vi "Describe Boolean Failure.vi"(1 "Expected":bool, 2 "Got":bool) -> (0 "Failure Description":string)   [LabVIEW 2013]
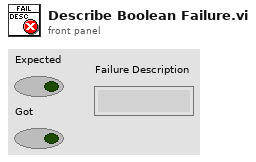
[diagram p1: front panel]
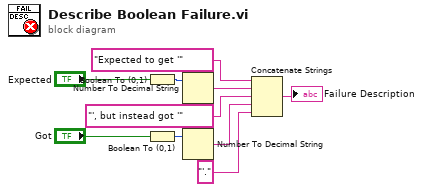
[diagram p0: block diagram]
diagram:
  n1 = Boolean To (0,1)(Boolean="Expected") -> (0, 1=w7:i16)
  n2 = Boolean To (0,1)(Boolean="Got") -> (0, 1=w8:i16)
  n3 = Number To Decimal String(number=w7) -> (decimal integer string=w5:string)  [unwired: 1 in]
  n4 = Number To Decimal String(number=w8) -> (decimal integer string=w2:string)  [unwired: 1 in]
  n5 = Concatenate Strings("Expected to get '", w5, "', but instead got '", w2, "'.") -> (→"Failure Description":string)
